vi "SAOMM-RaZ.vi"(0 "PRAMMS-COMM IN":refnum<visa-resource-name>="Hp\u0000\u0002", 1 "Active Refnum":refnum<vi>, 2 "PrAMS-ACK":refnum<vi>, 7 "Signature":u32=1886544237, 11 "Error IN":errorcluster, 12 "MessageType":cluster{string[], u32[]}={["emtError", "emtAreYouThere", "emtAcknowledgment", "emtGetClientType", "emtClientType", "emtGetImageExposureTime", "emtSetImageExposureTime", "emtImageExposureTime", "emtGetOptimalExposureTime", "emtSetOptimalExposureTime", "emtOptimalExposureTime", "emtGetImageEMGain", "emtSetImageEMGain", "emtImageEMGain", "emtGetFPGACtrl", "emtSetFPGACtrl", "emtFPGACtrl", "emtGetImageWidth", "emtSetImageWidth", "emtImageWidth", "emtGetImageHeight", "emtSetImageHeight", "emtImageHeight", "emtGetImageBinning", "emtSetImageBinning", "emtImageBinning", "emtGetImageDisplayFrameRate", "emtSetImageDisplayFrameRate", "emtImageDisplayFrameRate", "emtGetROIWidth", "emtSetROIWidth", "emtROIWidth", "emtGetROIHeight", "emtSetROIHeight", "emtROIHeight", "emtGetROIXOffset", "emtSetROIXOffset", "emtROIXOffset", "emtGetROIYOffset", "emtSetROIYOffset", "emtROIYOffset", "emtStartAcquisition", "mtStopAcquisition", "emtAcquisitionStarted", "emtAcquisitionStopped", "emtGetFalconImage", "emtFalconImage"], [1, 2, 3, 4, 5, 1001, 1101, 1201, 1002, 1102, 1202, 1003, 1103, 1203, 1004, 1104, 1204, 1005, 1105, 1205, 1006, 1106, 1206, 1007, 1107, 1207, 1008, 1108, 1208, 1009, 1109, 1209, 1010, 1110, 1210, 1011, 1111, 1211, 1012, 1112, 1212, 1130, 1131, 1150, 1151, 1070, 1270]}, 13 "Position U":dbl format="%.4f", 14 "Position V":dbl caption="Pos" format="%.4f") -> (4 "PRAMMS-COMM OUT":refnum<visa-resource-name>, 15 "Error OUT":errorcluster)   [LabVIEW 2019]
uses:
  Polymorphics/Num2littleEndian(DBL).vi
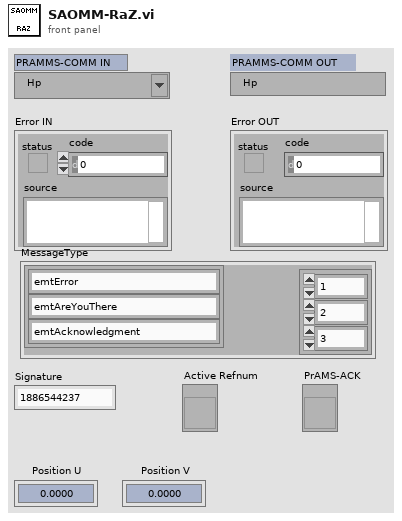
[diagram p1: front panel]
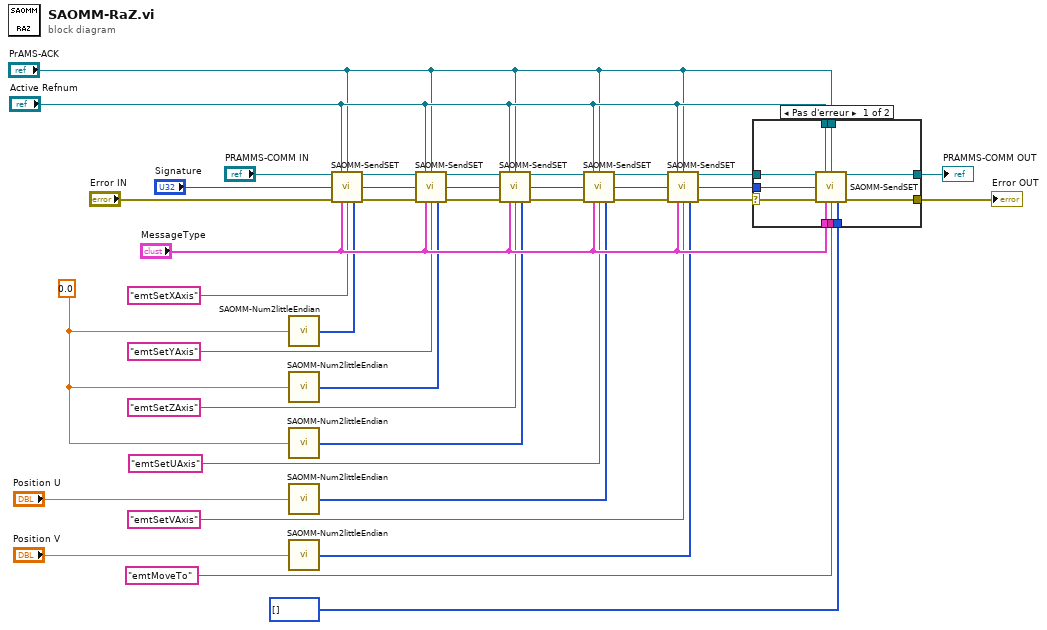
[diagram p0: block diagram]
diagram:
  w22 = 0.0
  n1 = call-poly "SAOMM-Num2littleEndian.vi"("Number"=w22) -> ("LiitleEndianedData"=w13:u8[])  [unwired: 14 in]
  n2 = call-poly "SAOMM-Num2littleEndian.vi"("Number"=w22) -> ("LiitleEndianedData"=w12:u8[])  [unwired: 14 in]
  n3 = call-poly "SAOMM-Num2littleEndian.vi"("Number"=w22) -> ("LiitleEndianedData"=w9:u8[])  [unwired: 14 in]
  n4 = call-poly "SAOMM-Num2littleEndian.vi"("Number"="Position U") -> ("LiitleEndianedData"=w7:u8[])  [unwired: 14 in]
  n5 = call-poly "SAOMM-Num2littleEndian.vi"("Number"="Position V") -> ("LiitleEndianedData"=w5:u8[])  [unwired: 14 in]
  n6 = call "SAOMM-SendSET.vi"("PRAMMS-COMM IN"="PRAMMS-COMM IN", "Active Refnum"="Active Refnum", "PrAMS-ACK"="PrAMS-ACK", "Signature"="Signature", "Error IN"="Error IN", "MessageType"="MessageType", "Active SET"="emtSetXAxis", "Value (little endianed byte array)"=w13) -> ("PRAMMS-COMM OUT"=w26:refnum<visa-resource-name>, "Error OUT"=w31:errorcluster)  [unwired: 4 in, 2 out]
  n7 = call "SAOMM-SendSET.vi"("PRAMMS-COMM IN"=w26, "Active Refnum"="Active Refnum", "PrAMS-ACK"="PrAMS-ACK", "Signature"="Signature", "Error IN"=w31, "MessageType"="MessageType", "Active SET"="emtSetYAxis", "Value (little endianed byte array)"=w12) -> ("PRAMMS-COMM OUT"=w27:refnum<visa-resource-name>, "Error OUT"=w30:errorcluster)  [unwired: 4 in, 2 out]
  n8 = call "SAOMM-SendSET.vi"("PRAMMS-COMM IN"=w27, "Active Refnum"="Active Refnum", "PrAMS-ACK"="PrAMS-ACK", "Signature"="Signature", "Error IN"=w30, "MessageType"="MessageType", "Active SET"="emtSetZAxis", "Value (little endianed byte array)"=w9) -> ("PRAMMS-COMM OUT"=w32:refnum<visa-resource-name>, "Error OUT"=w29:errorcluster)  [unwired: 4 in, 2 out]
  n9 = call "SAOMM-SendSET.vi"("PRAMMS-COMM IN"=w32, "Active Refnum"="Active Refnum", "PrAMS-ACK"="PrAMS-ACK", "Signature"="Signature", "Error IN"=w29, "MessageType"="MessageType", "Active SET"="emtSetUAxis", "Value (little endianed byte array)"=w7) -> ("PRAMMS-COMM OUT"=w33:refnum<visa-resource-name>, "Error OUT"=w28:errorcluster)  [unwired: 4 in, 2 out]
  n10 = call "SAOMM-SendSET.vi"("PRAMMS-COMM IN"=w33, "Active Refnum"="Active Refnum", "PrAMS-ACK"="PrAMS-ACK", "Signature"="Signature", "Error IN"=w28, "MessageType"="MessageType", "Active SET"="emtSetVAxis", "Value (little endianed byte array)"=w5) -> ("PRAMMS-COMM OUT"=w25:refnum<visa-resource-name>, "Error OUT"=w15:errorcluster)  [unwired: 4 in, 2 out]
  n11 = case shown="Pas d'erreur" w15 {
    selector: w15 -> [w38 w45]
    tunnel: w25 -> [w43 w44]
    tunnel: "Signature" -> [w42 _]
    tunnel: [w41 w44] -> w18
    tunnel: [w40 w45] -> w17
    tunnel: "MessageType" -> [w39 _]
    tunnel: "Active Refnum" -> [w37 _]
    tunnel: "PrAMS-ACK" -> [w36 _]
    tunnel: "emtMoveTo" -> [w35 _]
    tunnel: u8[] [] ("Value (little endianed byte array)") -> [w34 _]
    frame No Error {
      n12 = call "SAOMM-SendSET.vi"("PRAMMS-COMM IN"=w43, "Active Refnum"=w37, "PrAMS-ACK"=w36, "Signature"=w42, "Error IN"=w38, "MessageType"=w39, "Active SET"=w35, "Value (little endianed byte array)"=w34) -> ("PRAMMS-COMM OUT"=w41:refnum<visa-resource-name>, "Error OUT"=w40:errorcluster)  [unwired: 4 in, 2 out]
    }
    frame Error {
    }
  }
  "Error OUT" <- w17
  "PRAMMS-COMM OUT" <- w18
